vi "reportServerId.vi"(8 "error in (no error)":errorcluster, 11 "Subnet in":refnum<class "Subnet.lvclass">) -> (0 "error out":errorcluster, 3 "Subnet out":refnum<class "Subnet.lvclass">)   [LabVIEW 2016, in "Subnet.lvclass"]
uses:
  Subnet.lvclass
  Subnet.lvclass/Subnet.ctl
  Common_RT_HPILC/HPILC/HPILC.lvclass
  D:/Code/Common_RT_ILC/ILC/ILC.lvclass
  Common_RT_Modbus/IModbus/IModbus.lvclass
  Common_RT_ILC/ILC/ILC.lvclass
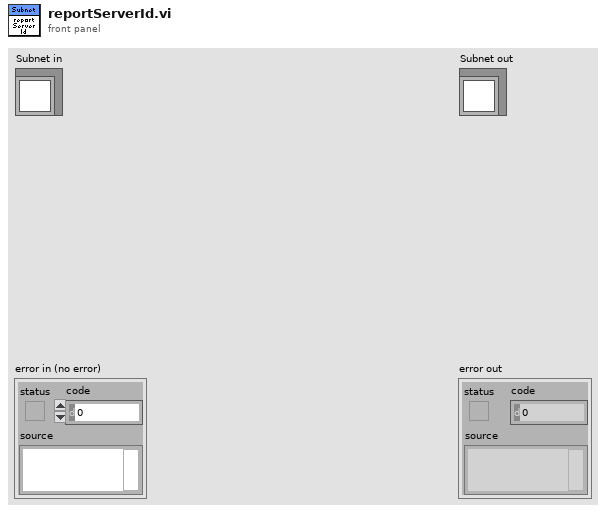
[diagram p1: front panel]
types:
  T1 = typedef "RTModbus.lvlib/TxFrame.ctl" = cluster{"Data":u8[], "WaitForTrigger":bool, "WaitForRx":u16, "TriggerIRQ":bool, "DelayMicroseconds":u16, "DelayMilliseconds":u16, "Timestamp":bool}
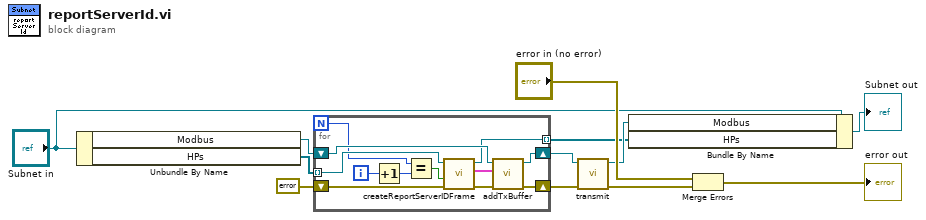
[diagram p0: block diagram]
diagram:
  n1 = Unbundle By Name("Subnet in") -> ("Modbus"=w10:refnum<class "IModbus.lvclass">, "HPs"=w6:refnum<class "HPILC.lvclass">[])
  n2 = for {
    N -> [w14]
    tunnel: w6 -> [w24] mode=indexing
    shift-right: [w22] -> w8
    shift-left: w10 -> [w23]
    shift-right: [w18] -> w7
    shift-left: errorcluster {"status"=FALSE, "code"=0, "source"=""} ("error out") -> [w19]
    tunnel: [w13] -> w2 mode=indexing
    i -> [w17]
    n3 = Increment(x=w17) -> (x+1=w16:i32)
    n4 = Equal?(x=w14, y=w16) -> (x = y?=w15:bool)
    n5 = call "createReportServerIDFrame.vi"("error in (no error)"=w19, "TriggerIRQ"=w15, "ILC in"=w24) -> ("error out"=w20:errorcluster, "TxFrame"=w21:T1, "ILC out"=w13:refnum<class "HPILC.lvclass">)  [unwired: 6 in]
    n6 = call-dynamic "addTxBuffer.vi"("error in (no error)"=w20, "TxFrame"=w21, "IModbus in"=w23) -> ("error out"=w18:errorcluster, "IModbus out"=w22:refnum<class "IModbus.lvclass">)  [unwired: 7 in]
  }
  n7 = call-dynamic "transmit.vi"("error in (no error)"=w7, "IModbus in"=w8) -> ("error out"=w1:errorcluster, "IModbus out"=w3:refnum<class "IModbus.lvclass">)  [unwired: 8 in]
  n8 = Bundle By Name(cluster="Subnet in", "Modbus"=w3, "HPs"=w2) -> (→"Subnet out":refnum<class "Subnet.lvclass">)
  n9 = Merge Errors("error in (no error)", w1) -> (→"error out":errorcluster)
